vi "SequenceIndicesTCShortcutMenuCreate.vi"(8 "error in (no error)":errorcluster, 10 "ShortcutMenuIn":T2, 11 "VMUI in":refnum<class "VMUI.lvclass">) -> (0 "error out":errorcluster, 2 "Discard?":bool, 3 "VMUI out":refnum<class "VMUI.lvclass">)   [LabVIEW 2013, in "VMUI.lvclass"]
uses:
  VMUI.lvclass
  <vilib>/Utility/miscctls.llb/LVPoint32TypeDef.ctl
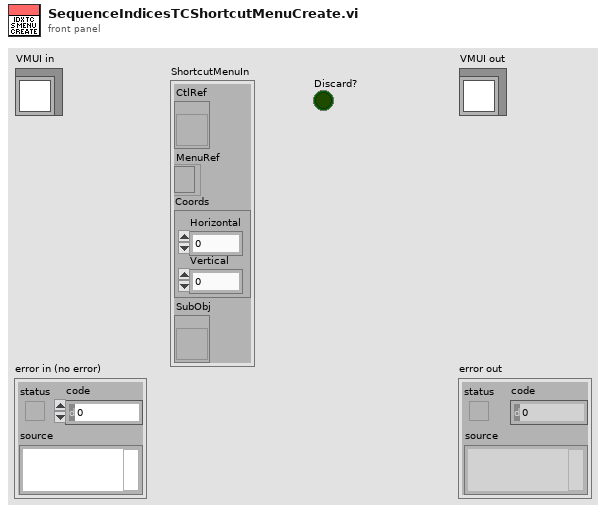
[diagram p1: front panel]
types:
  T1 = typedef "LVPoint32TypeDef.ctl" = cluster{"Horizontal":i32, "Vertical":i32}
  T2 = cluster{"CtlRef":refnum<vi>, "MenuRef":refnum<k9>, "Coords":T1, "SubObj":refnum<vi>}
  T3 = typedef "LVRowAndColumnTypeDef.ctl" = cluster{"Row":i32, "Column":i32}
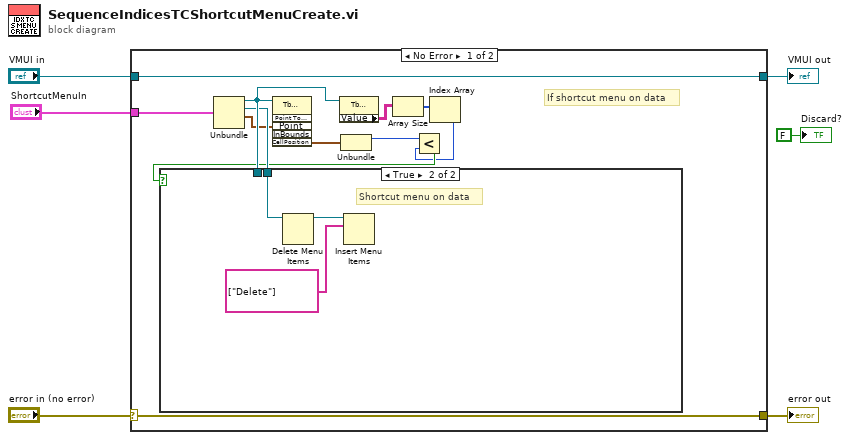
[diagram p0: block diagram]
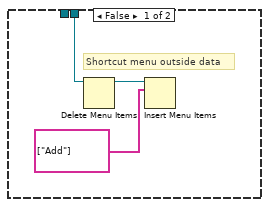
[diagram p2: hidden frame]
diagram:
  n1 = case shown="No Error" "error in (no error)" {
    selector: "error in (no error)" -> [w18 w26]
    tunnel: [w18 w26] -> w5
    tunnel: [w7 w25] -> w3
    tunnel: "VMUI in" -> [w7 w25]
    tunnel: "ShortcutMenuIn" -> [w10 _]
    frame No Error {
      # "If shortcut menu on data"
      n2 = Unbundle(w10) -> ("CtlRef"=w17:refnum<vi>, "MenuRef"=w16:refnum<k9>, "Coords"=w11:T1)  [unwired: 1 out]
      n3 = invoke class="Tbl (strict)" method="Point To Row Column"(reference=w17, "Point"=w11) -> ("CellPosition"=w14:T3)  [unwired: 4 in, 5 out]
      n4 = property class="Tbl (strict)"(reference=w17) -> ("Value"=w9:string[][])  [unwired: 1 in, 2 out]
      n5 = Unbundle(w14) -> ("Row"=w8:i32)  [unwired: 1 out]
      n6 = Array Size(array=w9) -> (size(s)=w13:i32[])
      n7 = Index Array(array=w13) -> (element=w12:i32)  [unwired: 1 in]
      n8 = Less?(x=w8, y=w12) -> (x < y?=w15:bool)
      n9 = case shown="True" w15 {
        tunnel: w16 -> [w21 w23]
        tunnel: w17 -> [_ _]
        frame False {
          # "Shortcut menu outside data"
          n10 = Delete Menu Items(9:w21) -> (3:w20:refnum<k9>)  [unwired: 3 in, 1 out]
          n11 = Insert Menu Items(8:string[] ["Add"] ("item names"), 9:w20) -> ()  [unwired: 4 in, 3 out]
        }
        frame True {
          # "Shortcut menu on data"
          n12 = Delete Menu Items(9:w23) -> (3:w24:refnum<k9>)  [unwired: 3 in, 1 out]
          n13 = Insert Menu Items(8:string[] ["Delete"] ("item names"), 9:w24) -> ()  [unwired: 4 in, 3 out]
        }
      }
    }
    frame Error {
    }
  }
  "error out" <- w5
  "VMUI out" <- w3
  "Discard?" <- FALSE ("Discard?")
